vi "Generate Search ID.vi"(11 "Search":refnum<class "Search.lvclass">) -> (3 "Search ID":string)   [LabVIEW 2016, in "Better Search.lvlib" / "BetterSearch.lvclass"]
uses:
  BetterSearch.lvclass
  Search/Search.lvclass
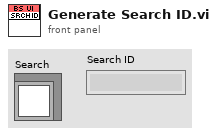
[diagram p1: front panel]
types:
  T1 = typedef "Better Search.lvlib/Search Params.ctl" = cluster{"Type":T2, "Type ID":string, "Text":string, "Scope":T3, "Targets":refnum<vi>[], "Scope Options":T4, "Typedef Path":path, "Member Graph Index":i32, "Member TypeID":string}
  T2 = typedef "Better Search.lvlib/Search Type.ctl" = enum16{"Generic", "Text", "Data Type", "VI", "Node"}
  T3 = typedef "Better Search.lvlib/Search Scope.ctl" = enum16{"Active Target", "Active Project", "Specific Targets", "Active VI", "Active Hierarchy"}
  T4 = typedef "Better Search.lvlib/Scope Options.ctl" = cluster{"Include Labels":bool, "Include Captions":bool, "Include Node Name":bool, "Member Access":bool, "Member Read":bool, "Member Write":bool, "Member Name":string, "String Value":bool, "Dependencies":bool, "vi.lib":bool, "user.lib":bool, "instr.lib":bool}
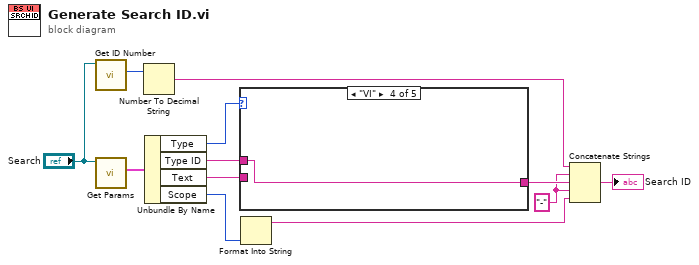
[diagram p0: block diagram]
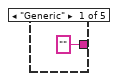
[diagram p2: hidden frame]
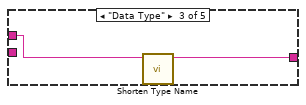
[diagram p4: hidden frame]
diagram:
  w4 = "-" ("string")
  n1 = call "Get ID Number.vi"("Search in"="Search") -> ("ID #"=w2:i32)  [unwired: 8 in, 2 out]
  n2 = call "Get Params.vi"("Search in"="Search") -> ("Params"=w12:T1)  [unwired: 8 in, 2 out]
  n3 = Number To Decimal String(number=w2) -> (decimal integer string=w1:string)  [unwired: 1 in]
  n4 = Unbundle By Name(w12) -> ("Type"=w10:T2, "Type ID"=w9:string, "Text"=w8:string, "Scope"=w11:T3)
  n5 = case shown="\"VI\"" w10 {
    tunnel: w9 -> [_ _ w15 w17 w18]
    tunnel: w8 -> [_ w14 _ _ _]
    tunnel: ["" ("Style") w14 w16 w17 w18] -> w5
    frame "Generic" {
    }
    frame "Text" {
    }
    frame "Data Type" {
      n6 = call "Shorten Type Name.vi"("Name In"=w15) -> ("Limited Name"=w16:string)  [unwired: 10 in]
    }
    frame "VI" {
    }
    frame "Node" {
    }
  }
  n7 = Format Into String(w11) -> (resulting string=w7:string)  [unwired: 3 in, 1 out]
  n8 = Concatenate Strings(w1, w4, w5, w4, w7) -> (→"Search ID":string)
